vi "Pin Configuration Reset.vi"(8 "error in":errorcluster, 11 "Handle In":i32) -> (0 "error out":errorcluster, 3 "Handle Out":i32)   [LabVIEW 2021]
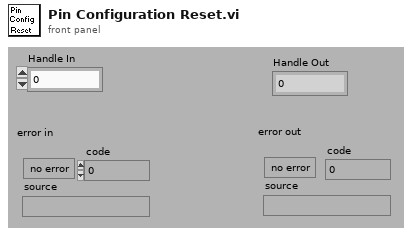
[diagram p1: front panel]
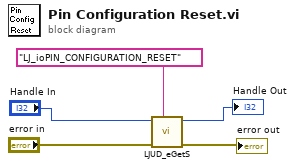
[diagram p0: block diagram]
diagram:
  n1 = call "LJUD_eGetS.vi"("IOType"="LJ_ioPIN_CONFIGURATION_RESET", "error in"="error in", "Handle In"="Handle In") -> ("error out"=→"error out":errorcluster, "Handle Out"=→"Handle Out":i32)  [unwired: 6 in, 1 out]
